vi "stop-all-axis-amit.vi"(8 "error in (no error)":errorcluster) -> (0 "error out":errorcluster, 3 "Status":u32)   [LabVIEW 2009]
panel:
  # "PI"
  # "C844 STOP ALL"
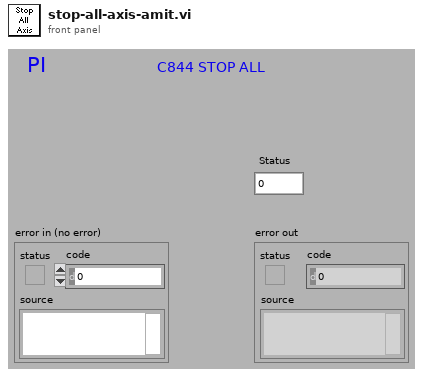
[diagram p1: front panel]
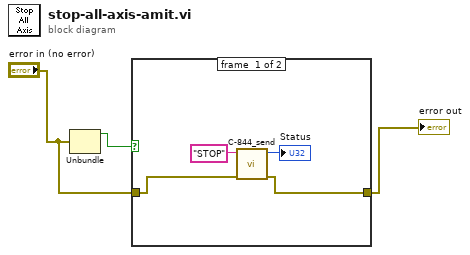
[diagram p0: block diagram]
diagram:
  n1 = Unbundle("error in (no error)") -> ("status"=w3:bool)  [unwired: 2 out]
  n2 = case shown="False" w3 {
    tunnel: "error in (no error)" -> [w7 w8]
    tunnel: [w6 w8] -> w1
    frame #0 {
      n3 = call "C-844_send.vi"("error in (no error)"=w7, "Command"="STOP") -> ("error out"=w6:errorcluster, "Status"=→"Status":u32)  [unwired: 7 in, 1 out]
    }
    frame #1 {
    }
  }
  "error out" <- w1
